vi "RaceCondition.vi"() -> ()   [LabVIEW 2020]
panel:
  in  "Numeric":dbl
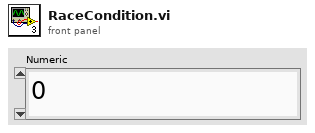
[diagram p1: front panel]
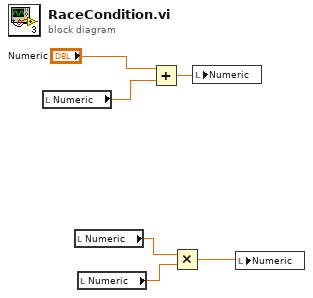
[diagram p0: block diagram]
diagram:
  n1 = local read "Numeric"() -> (w5:dbl)
  n2 = local read "Numeric"() -> (w3:dbl)
  n3 = local read "Numeric"() -> (w2:dbl)
  n4 = Add(x="Numeric", y=w5) -> (x+y=w4:dbl)
  n5 = Multiply(x=w3, y=w2) -> (x*y=w1:dbl)
  n6 = local write "Numeric"(w4) -> ()
  n7 = local write "Numeric"(w1) -> ()
